vi "FormulaNode_Ejemplo.vi"() -> ()   [LabVIEW 2022 SP3]
panel:
  in  "stop":bool
  out "Fahrenheit":dbl
  in  "Celsius":dbl
  # "F=9*C/5+32"
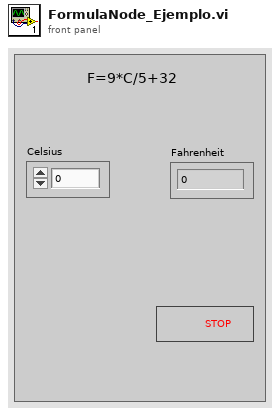
[diagram p1: front panel]
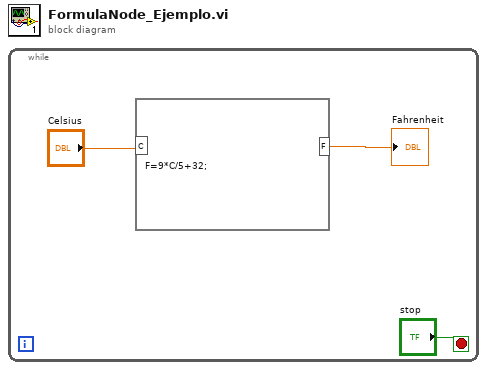
[diagram p0: block diagram]
diagram:
  n1 = while {
    stop <- "stop" stop-if-true
    n2 = formula code="F=9*C/5+32;"("C"="Celsius") -> ("F"=→"Fahrenheit":dbl)
  }
